vi "AlliGator Save-Load Phasor Color Map.vi"(6 "Save/Load (F)":bool, 8 "Error In":errorcluster, 11 "Control References":T1) -> (0 "Error Out":errorcluster)   [LabVIEW 2021, in "AlliGator Phasor Plot Color Map.lvlib"]
doc: "Saves/Loads a Phasor Plot Color Map from a XML file."
uses:
  AlliGator Phasor Plot Color Map.lvlib
  AlliGator Phasor Color Map Definition.ctl
  <vilib>/Utility/miscctls.llb/LVCursorListTypeDef.ctl
  Files/Files.lvlib
panel:
  # "see the AlliGator License on the block diagram (Ctrl+E or Window:Show Block Diagram)"
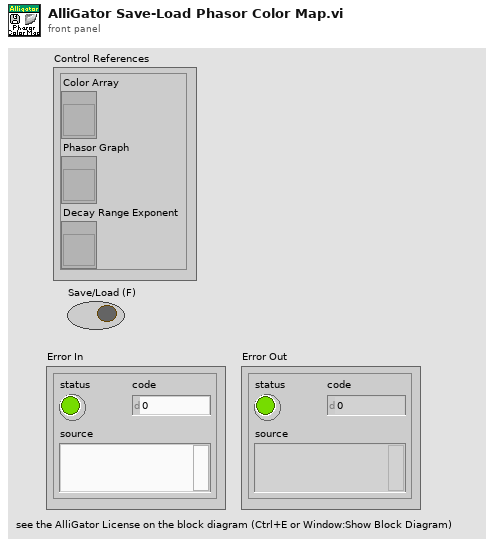
[diagram p1: front panel]
types:
  T1 = cluster{"Color Array":refnum<vi>, "Phasor Graph":refnum<vi>, "Decay Range Exponent":refnum<vi>}
  T2 = typedef "AlliGator Phasor Plot Color Map.lvlib/AlliGator Phasor Color Map Definition.ctl" = cluster{"Color Array":u32[], "Cursor Array":T3, "Decay Range Exponent":dbl}
  T3 = typedef "LVCursorListTypeDef.ctl" = cluster{"Name":string, "Color":u32, "Style":u8, "Point Style":u8, "Name Visible":bool, "Allow Drag":bool, "Cursor Mode":u32, "Plot":i32, "Index":i32, "Position":cluster{"X":dbl, "Y":dbl}, "X Scale":u32, "Y Scale":u32, "Watch Plots":i32[], "Watch All Plots":bool, "Plot Area":i32, "Label Offset":cluster{"X":dbl, "Y":dbl}}[]
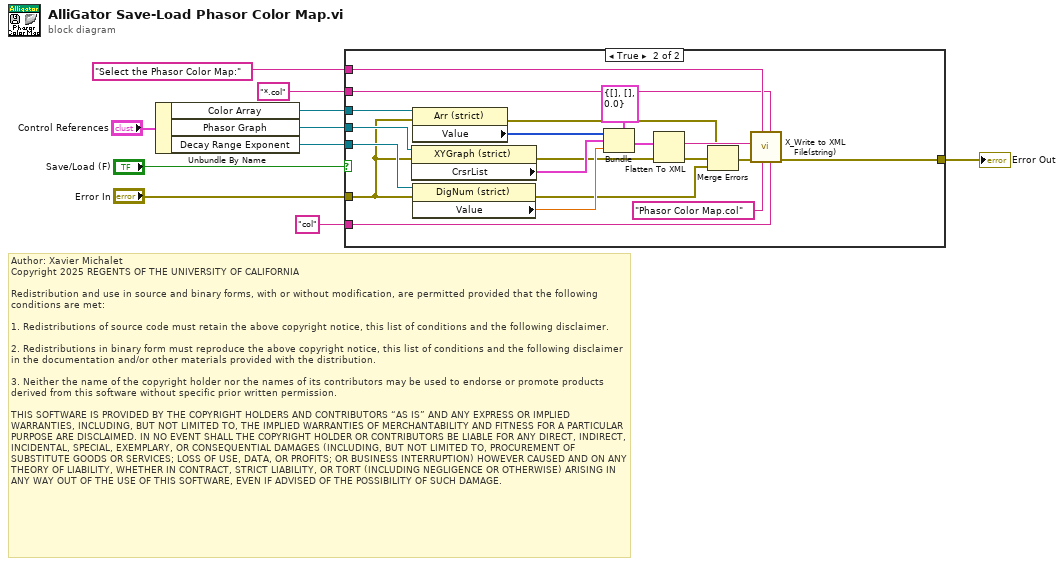
[diagram p0: block diagram]
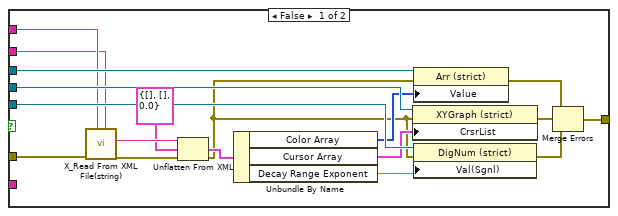
[diagram p2: hidden frame]
diagram:
  # "Author: Xavier Michalet\nCopyright 2025 REGENTS OF THE UNIVERSITY OF CALIFORNIA\n\nRedistribution and use in source and binary forms, with or without modification, are permitted provided that the following conditions are met:\n\n1. Redistributions of source code must retain the above copyright notice, this list of conditions and the following disclaimer.\n\n2. Redistributions in binary form must reproduce the above copyright notice, this list of conditions and the following disclaimer in the documentation and/or other materials provided with the distribution.\n\n3. Neither the name of the copyright holder nor the names of its contributors may be used to endorse or promote products derived from this software without specific prior written permission.\n\nTHIS SOFTWARE IS PROVIDED BY THE COPYRIGHT HOLDERS AND CONTRIBUTORS “AS IS” AND ANY EXPRESS OR IMPLIED WARRANTIES, INCLUDING, BUT NOT LIMITED TO, THE IMPLIED WARRANTIES OF MERCHANTABILITY AND FITNESS FOR A PARTICULAR PURPOSE ARE DISCLAIMED. IN NO EVENT SHALL THE COPYRIGHT HOLDER OR CONTRIBUTORS BE LIABLE FOR ANY DIRECT, INDIRECT, INCIDENTAL, SPECIAL, EXEMPLARY, OR CONSEQUENTIAL DAMAGES (INCLUDING, BUT NOT LIMITED TO, PROCUREMENT OF SUBSTITUTE GOODS OR SERVICES; LOSS OF USE, DATA, OR PROFITS; OR BUSINESS INTERRUPTION) HOWEVER CAUSED AND ON ANY THEORY OF LIABILITY, WHETHER IN CONTRACT, STRICT LIABILITY, OR TORT (INCLUDING NEGLIGENCE OR OTHERWISE) ARISING IN ANY WAY OUT OF THE USE OF THIS SOFTWARE, EVEN IF ADVISED OF THE POSSIBILITY OF SUCH DAMAGE."
  n1 = Unbundle By Name("Control References") -> ("Color Array"=w9:refnum<vi>, "Phasor Graph"=w8:refnum<vi>, "Decay Range Exponent"=w7:refnum<vi>)
  n2 = case shown="True" "Save/Load (F)" {
    tunnel: w9 -> [w28 w47]
    tunnel: w8 -> [w27 w46]
    tunnel: w7 -> [w26 w45]
    tunnel: "Error In" -> [w22 w38]
    tunnel: [w17 w33] -> w5
    tunnel: "Select the Phasor Color Map:" ("Prompt") -> [w12 w32]
    tunnel: "*.col" ("Pattern (*.xml;*.XML)") -> [w11 w31]
    tunnel: "col" ("File Extension (xml)") -> [_ w30]
    frame False {
      n3 = call "X_Read From XML File(string).vi"("pattern (*.xml)"=w11, "Prompt"=w12, "error in (no error)"=w22) -> ("error out"=w20:errorcluster, "XML Elements"=w21:string)  [unwired: 6 in, 1 out]
      n4 = Unflatten From XML(xml string=w21, type=T2 {"Color Array"=[], "Cursor Array"=[], "Decay Range Exponent"=0.0} ("cluster"), error in (no error)=w20) -> (value=w18:T2, error out=w13:errorcluster)
      n5 = Unbundle By Name(w18) -> ("Color Array"=w16:u32[], "Cursor Array"=w15:T3, "Decay Range Exponent"=w14:dbl)
      n6 = property class="XYGraph (strict)"(reference=w27, error in=w13, "CrsrList"=w15) -> (error out=w24:errorcluster)  [unwired: 1 out]
      n7 = property class="Arr (strict)"(reference=w28, error in=w13, "Value"=w16) -> (error out=w25:errorcluster)  [unwired: 1 out]
      n8 = property class="DigNum (strict)"(reference=w26, error in=w13, "Val(Sgnl)"=w14) -> (error out=w23:errorcluster)  [unwired: 1 out]
      n9 = Merge Errors(w25, w24, w23) -> (w17:errorcluster)
    }
    frame True {
      n10 = property class="XYGraph (strict)"(reference=w46, error in=w38) -> (error out=w36:errorcluster, "CrsrList"=w43:T3)  [unwired: 1 out]
      n11 = property class="Arr (strict)"(reference=w47, error in=w38) -> (error out=w37:errorcluster, "Value"=w44:u32[])  [unwired: 1 out]
      n12 = property class="DigNum (strict)"(reference=w45, error in=w38) -> (error out=w35:errorcluster, "Value"=w42:dbl)  [unwired: 1 out]
      n13 = Bundle(cluster=T2 {"Color Array"=[], "Cursor Array"=[], "Decay Range Exponent"=0.0}, "Color Array"=w44, "Cursor Array"=w43, "Decay Range Exponent"=w42) -> (w40:T2)
      n14 = Flatten To XML(6:w40) -> (2:w39:string)
      n15 = Merge Errors(w37, w36, w35) -> (w34:errorcluster)
      n16 = call "X_Write to XML File(string).vi"("File Extension (xml)"=w30, "Pattern (*.xml;*.XML)"=w31, "default name"="Phasor Color Map.col", "Prompt"=w32, "error in (no error)"=w34, "XML Input"=w39) -> ("error out"=w33:errorcluster)  [unwired: 2 in, 3 out]
    }
  }
  "Error Out" <- w5
